vi "launch.vi"(8 "error in (no error)":errorcluster, 11 "TaskController in":refnum<class "TaskController.lvclass">) -> (0 "error out":errorcluster, 3 "TaskController out":refnum<class "TaskController.lvclass">)   [LabVIEW 2023, in "TLC_Daemon.lvlib" / "TaskController.lvclass"]
doc: "Launches the task."
uses:
  TaskController.lvclass
  TaskController.lvclass/TaskController.ctl
  status.ctl
  ITask/ITask.lvclass
  ITaskChannel/ITaskChannel.lvclass
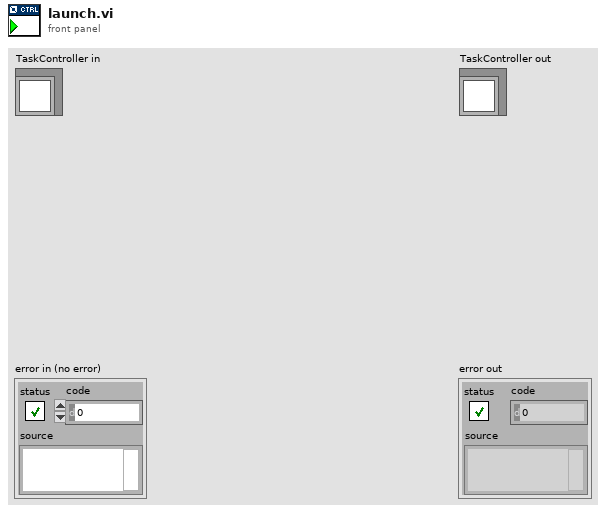
[diagram p1: front panel]
types:
  T1 = typedef "TLC_Daemon.lvlib/TaskController.lvclass/status.ctl" = enum16{"NotReady", "Ready", "Running", "Stopped", "Unknown"}
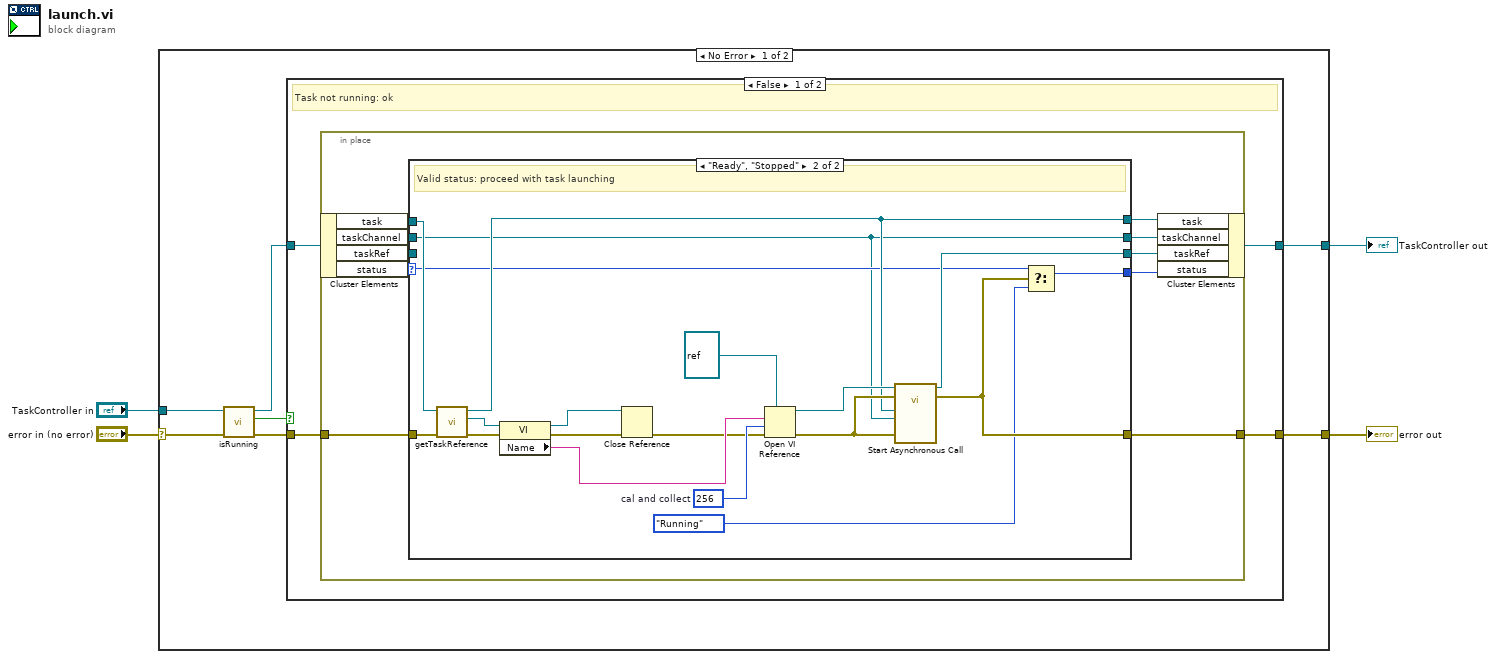
[diagram p0: block diagram]
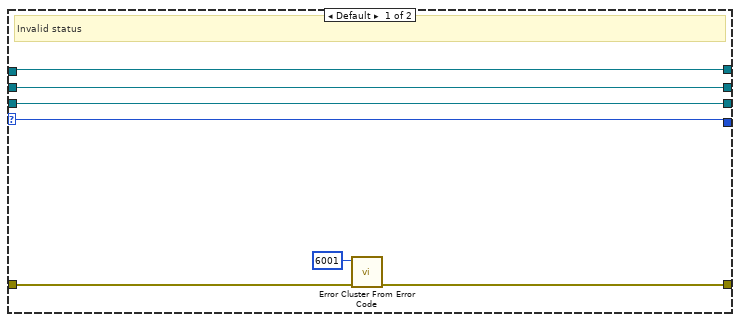
[diagram p2: hidden frame]
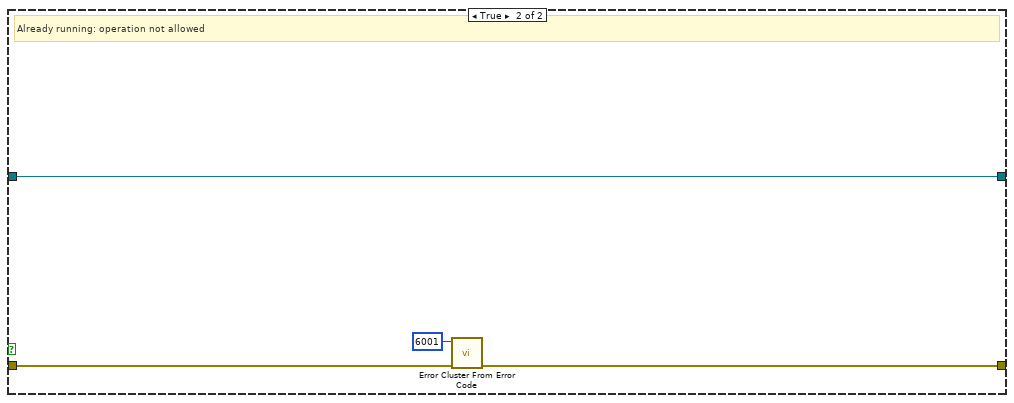
[diagram p3: hidden frame]
diagram:
  n1 = case shown="No Error" "error in (no error)" {
    selector: "error in (no error)" -> [w9 w57]
    tunnel: [w11 w57] -> w3
    tunnel: [w10 w56] -> w1
    tunnel: "TaskController in" -> [w6 w56]
    frame No Error {
      n2 = call "isRunning.vi"("error in (no error)"=w9, "TaskController in"=w6) -> ("error out"=w8:errorcluster, "isRunning"=w5:bool, "TaskController out"=w7:refnum<class "TaskController.lvclass">)  [unwired: 7 in]
      n3 = case shown="False" w5 {
        tunnel: [w15 w53] -> w11
        tunnel: [w14 w55] -> w10
        tunnel: w8 -> [w13 w52]
        tunnel: w7 -> [w12 w55]
        frame False {
          # "Task not running: ok"
          n4 = in-place {
            in-place-border: w13 -> [w25]
            in-place-border: [w21] -> w15
            n5 = in-place-cluster #1(w12) -> ("task"=w23:refnum<class "ITask.lvclass">, "taskChannel"=w17:refnum<class "ITaskChannel.lvclass">, "taskRef"=w18:refnum<vi>, "status"=w20:T1)
            n6 = case shown="\"Ready\", \"Stopped\"" w20 {
              selector: w20 -> [w32 w36]
              tunnel: w25 -> [w27 w51]
              tunnel: [w31 w43] -> w24
              tunnel: w23 -> [w29 w39]
              tunnel: [w29 w38] -> w22
              tunnel: [w28 w37] -> w21
              tunnel: [w32 w35] -> w19
              tunnel: w18 -> [w31 _]
              tunnel: w17 -> [w30 w33]
              tunnel: [w30 w33] -> w16
              frame Default {
                # "Invalid status"
                n7 = call <vilib>:"Error Cluster From Error Code.vi"("error in (no error)"=w27, "error code (0)"=6001) -> ("error out"=w28:errorcluster)  [unwired: 7 in]
              }
              frame "Ready", "Stopped" {
                w50 = 256  # cal and collect
                # "Valid status: proceed with task launching"
                n8 = call-dynamic "getTaskReference.vi"("error in (no error)"=w51, "ITask in"=w39) -> ("error out"=w44:errorcluster, "taskRef"=w46:refnum<vi>, "ITask out"=w38:refnum<class "ITask.lvclass">)  [unwired: 7 in]
                n9 = property class="VI"(reference=w46, error in=w44) -> (reference out=w40:refnum<vi>, error out=w42:errorcluster, "Name"=w45:string)
                n10 = Close Reference(reference=w40, error in (no error)=w42) -> (error out=w41:errorcluster)
                n11 = Open VI Reference(type specifier VI Refnum (for type only)=refnum<vi> refnum, vi path=w45, options=w50, error in (no error)=w41) -> (vi reference=w48:refnum<vi>, error out=w47:errorcluster)  [unwired: 2 in]
                n12 = call-by-ref "Start Asynchronous Call"(reference=w48, error in=w47, 8:"error in (no error)"=w47, "stopMechanism"=w33, "ITask in"=w38) -> (reference out=w43:refnum<vi>, error out=w37:errorcluster)  [unwired: 7 in, 2 out]
                n13 = Select(t=w36, s=w37, f=status."Running") -> (s? t:f=w35:T1)
              }
            }
            n14 = in-place-cluster #1("task"=w22, "taskChannel"=w16, "taskRef"=w24, "status"=w19) -> (w14:refnum<class "TaskController.lvclass">)
          }
        }
        frame True {
          # "Already running: operation not allowed"
          n15 = call <vilib>:"Error Cluster From Error Code.vi"("error in (no error)"=w52, "error code (0)"=6001) -> ("error out"=w53:errorcluster)  [unwired: 7 in]
        }
      }
    }
    frame Error {
    }
  }
  "error out" <- w3
  "TaskController out" <- w1
